vi "ScanFromString2.vi"() -> ()   [LabVIEW 2019]
panel:
  out "salary o/p":u32
  out "age o/p":u8
  out "name o/p":string
  in  "Input String":string="Name of Employee is Atul . His age is 29 and He receives salary of 10000000"
  out "String":string
  in  "salary":u32=10000000
  in  "age":u8=29
  in  "name":string="Atul"
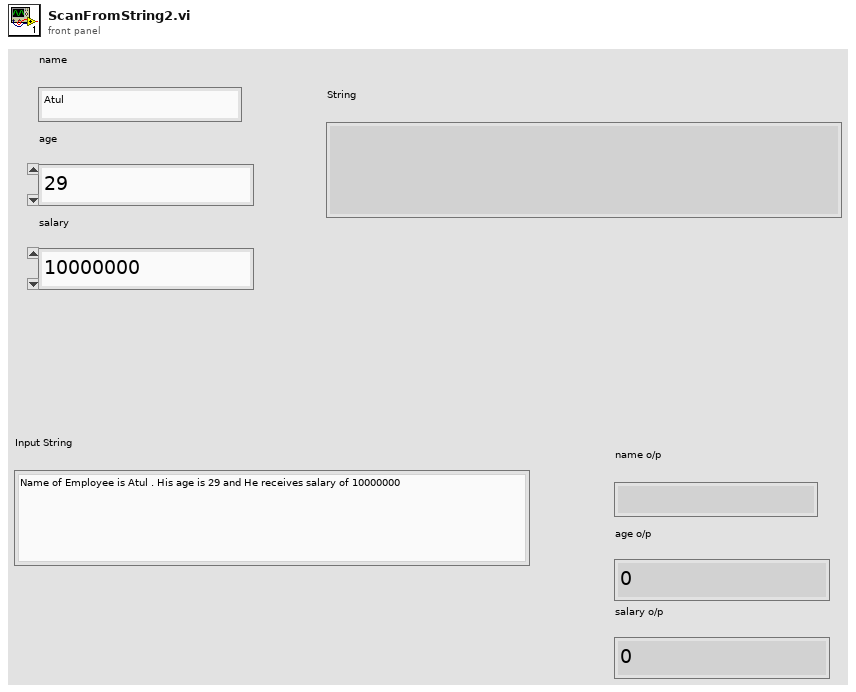
[diagram p1: front panel]
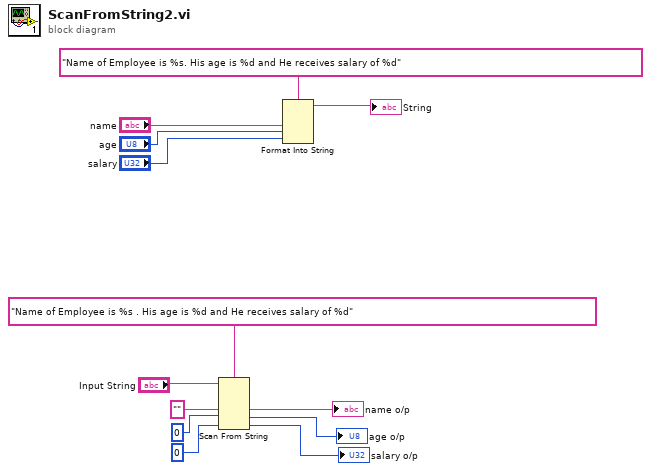
[diagram p0: block diagram]
diagram:
  n1 = Scan From String(format string="Name of Employee is %s . His age is %d and He receives salary of %d", input string="Input String", default 1="" ("default value 1"), default 2=u8 0, default 3=u32 0) -> (output 1=→"name o/p":string, output 2=→"age o/p":u8, output 3=→"salary o/p":u32)  [unwired: 2 in, 3 out]
  n2 = Format Into String(format string="Name of Employee is %s. His age is %d and He receives salary of %d", "name", "age", "salary") -> (resulting string=→"String":string)  [unwired: 2 in, 1 out]
